vi "Get Windows Process Memory Usage.vi"(8 "Error In":errorcluster) -> (0 "Error Out":errorcluster, 1 "Process Summary":string[][](table), 2 "Labview StartTime":timestamp, 3 "Memory Used By This Process - Labview (KB)":dbl, 4 "Memory Usage Total (KB)":i64, 6 "Number of processes":i32)   [LabVIEW 2017]
panel:
  out "Process Name":string[](array[string])
  out "Process ID":i32[](array[numeric])
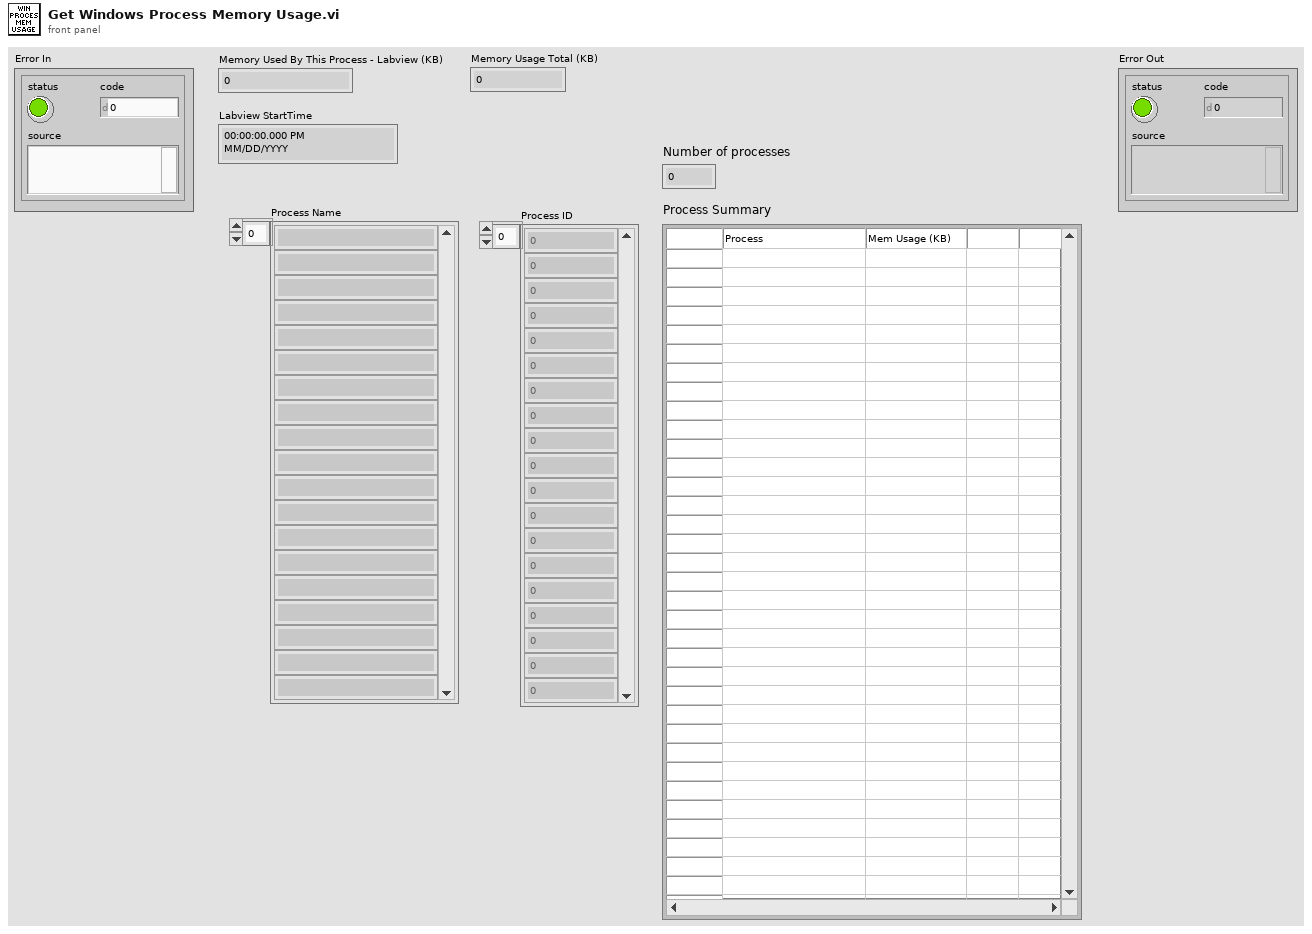
[diagram p1: front panel]
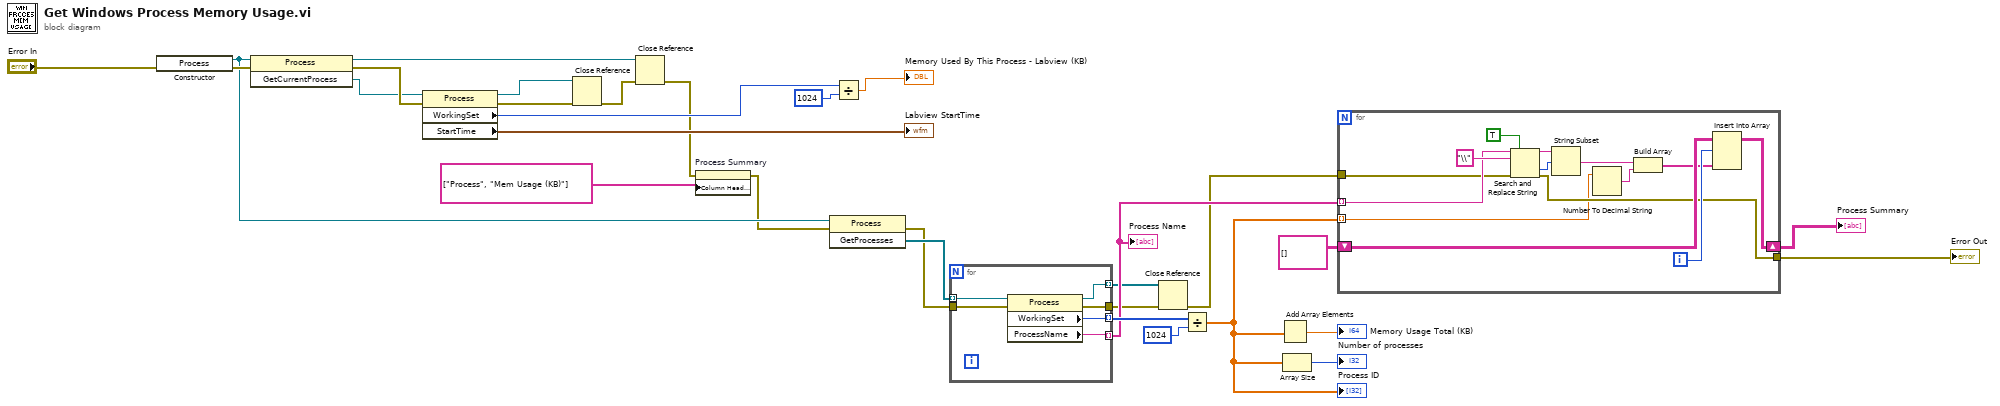
[diagram p0: block diagram]
diagram:
  n1 = constructor class="Process"(error in="Error In") -> (reference out=w10:refnum<k24>, error out=w23:errorcluster)  [unwired: 2 in, 1 out]
  n2 = invoke class="Process" method="GetCurrentProcess"(reference=w10, error in=w23) -> (reference out=w9:refnum<k24>, error out=w30:errorcluster, "GetCurrentProcess"=w8:refnum<k24>)  [unwired: 1 in]
  n3 = property class="Process"(reference=w8, error in=w30) -> (reference out=w27:refnum<k24>, error out=w26:errorcluster, "WorkingSet"=w24:i32, "StartTime"=→"Labview StartTime":timestamp)
  n4 = Close Reference(reference=w27, error in (no error)=w26) -> (error out=w28:errorcluster)
  n5 = Close Reference(reference=w9, error in (no error)=w28) -> (error out=w1:errorcluster)
  n6 = property on="Process Summary" class="Tbl (strict)"(error in=w1, "Column Header Strings[]"=string[] ["Process", "Mem Usage (KB)"] ("new element/subarray")) -> (error out=w2:errorcluster)  [unwired: 1 in, 1 out]
  n7 = invoke class="Process" method="GetProcesses"(reference=w10, error in=w2) -> (error out=w4:errorcluster, "GetProcesses"=w22:refnum<k24>[])  [unwired: 1 in, 1 out]
  n8 = Divide(x=w24, y=i64 1024) -> (x/y=→"Memory Used By This Process - Labview (KB)":dbl)
  n9 = for {
    tunnel: w22 -> [w36] mode=indexing
    tunnel: [w35] -> w20 mode=indexing
    tunnel: [w34] -> w14 mode=indexing
    tunnel: [w33] -> w11 mode=indexing
    tunnel: [w32] -> w5
    tunnel: w4 -> [w31]
    n10 = property class="Process"(reference=w36, error in=w31) -> (reference out=w33:refnum<k24>, error out=w32:errorcluster, "WorkingSet"=w35:i32, "ProcessName"=w34:string)
  }
  "Process Name" <- w14
  n11 = Close Reference(reference=w11, error in (no error)=w5) -> (error out=w3:errorcluster)
  n12 = Divide(x=w20, y=i64 1024) -> (x/y=w13:dbl[])
  "Process ID" <- w13
  n13 = Add Array Elements(numeric array=w13) -> (sum=→"Memory Usage Total (KB)":dbl)
  n14 = Array Size(array=w13) -> (size(s)=→"Number of processes":i32)
  n15 = for {
    tunnel: w14 -> [w46] mode=indexing
    shift-right: [w40] -> w16
    shift-left: string[][] [] ("Process Summary") -> [w42]
    tunnel: w3 -> [w39]
    tunnel: [w38] -> w6
    tunnel: w13 -> [w37] mode=indexing
    i -> [w43]
    n16 = Search and Replace String(replace all?=TRUE ("replace all? (F)"), input string=w46, search string="\\", error in=w39) -> (result string=w44:string, offset past replacement=w47:i32, error out=w38:errorcluster)  [unwired: 4 in, 1 out]
    n17 = String Subset(string=w44, offset (0)=w47) -> (substring=w45:string)  [unwired: 1 in]
    n18 = Number To Decimal String(number=w37) -> (decimal integer string=w50:string)  [unwired: 1 in]
    n19 = Build Array(w45, w50) -> (w41:string[])
    n20 = Insert Into Array(array=w42, index (row)=w43, new element=w41) -> (w40:string[][])  [unwired: 1 in]
  }
  "Process Summary" <- w16
  "Error Out" <- w6
